vi "Destroy TimerDRV.vi"(8 "error in (no error)":errorcluster, 11 "TimerDRV in":refnum<class "TimerDRV.lvclass">) -> (0 "error out":errorcluster)   [LabVIEW 2019, in "TimingDRV Engine.lvlib" / "TimerDRV.lvclass"]
uses:
  TimerDRV.lvclass
  TimerDRV.lvclass/TimerDRV.ctl
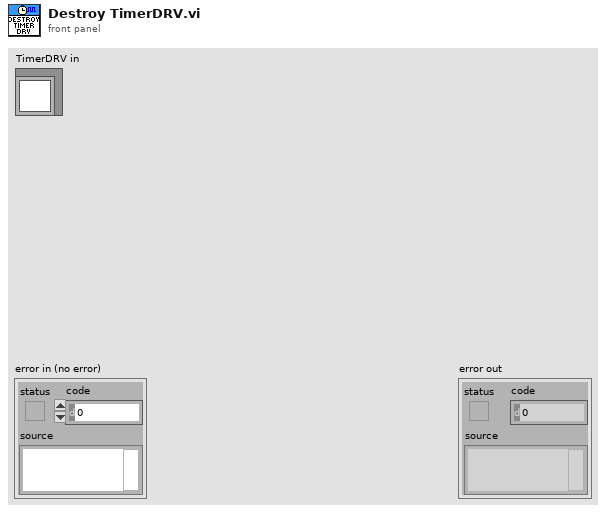
[diagram p1: front panel]
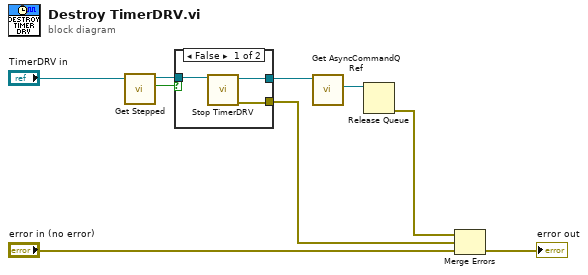
[diagram p0: block diagram]
diagram:
  n1 = call "Get Stepped.vi"("TimerDRV in"="TimerDRV in") -> ("Stepped"=w1:bool, "TimerDRV out"=w2:refnum<class "TimerDRV.lvclass">)  [unwired: 9 in]
  n2 = case shown="False" w1 {
    tunnel: [w12 w13] -> w6
    tunnel: [w11 _] -> w4
    tunnel: w2 -> [w10 w13]
    frame False {
      n3 = call "Stop TimerDRV.vi"("TimerDRV in"=w10) -> ("error out"=w11:errorcluster, "TimerDRV out"=w12:refnum<class "TimerDRV.lvclass">)  [unwired: 9 in]
    }
    frame True {
    }
  }
  n4 = call "Get AsyncCommandQ Ref.vi"("TimerDRV in"=w6) -> ("AsyncCommandQ"=w7:refnum<queue>)  [unwired: 9 in, 1 out]
  n5 = Release Queue(queue=w7) -> (error out=w5:errorcluster)  [unwired: 2 in, 2 out]
  n6 = Merge Errors(w5, w4, "error in (no error)") -> (→"error out":errorcluster)
